vi "from string.vi"(8 "error in":errorcluster, 9 "channel data":string, 10 "identifier":string, 11 "channel in":refnum<class "fpga channel.lvclass">) -> (0 "error out":errorcluster, 3 "channel out":refnum<class "fpga channel.lvclass">)   [LabVIEW 2015, in "fpga channel.lvclass"]
uses:
  fpga channel.lvclass
  fpga channel.lvclass/fpga channel.ctl
  Read FXP type.vi
  Write FXP type.vi
  <vilib>/NI/Tag Bus Module Framework/channel/TBM channel.lvclass
  <vilib>/NI/Configuration Framework/serializable configuration/NISE_CEF_serializable configuration.lvclass
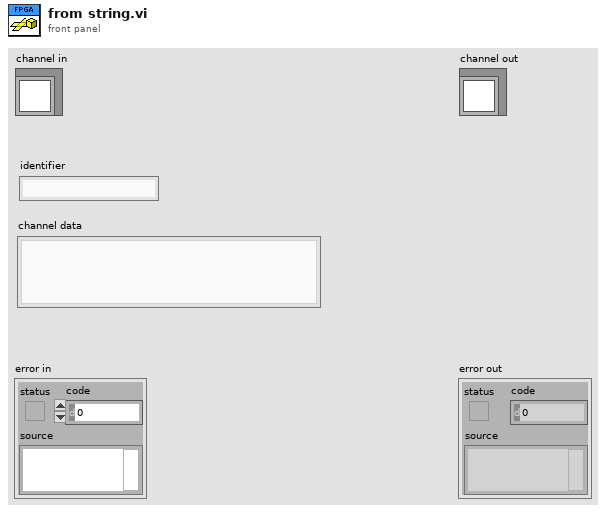
[diagram p1: front panel]
types:
  T1 = typedef "LVFixedPointRepBitsTypeDef.ctl" = cluster{"Signed":bool, "Word Length":u32, "Integer Word Length":i32}
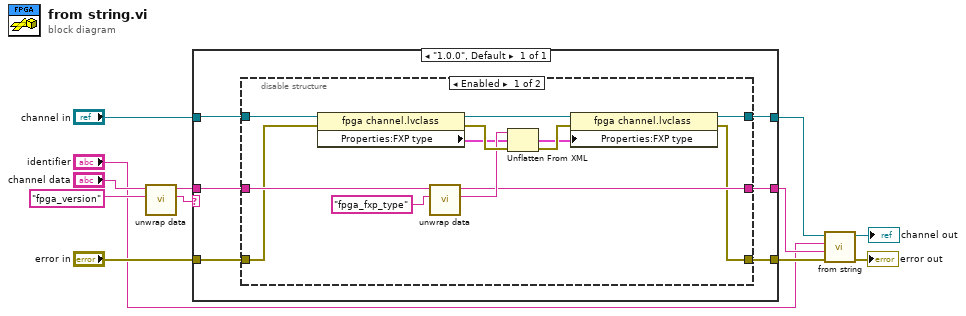
[diagram p0: block diagram]
diagram:
  n1 = call <vilib>:"unwrap data.vi"("identifier"="fpga_version", "data to unwrap"="channel data") -> ("unwrapped data"=w6:string, "remaining string"=w7:string)  [unwired: 8 in]
  n2 = case shown="\"1.0.0\", Default" w6 {
    tunnel: "error in" -> [w15]
    tunnel: w7 -> [w17]
    tunnel: "channel in" -> [w14]
    tunnel: [w18] -> w4
    tunnel: [w16] -> w3
    tunnel: [w13] -> w2
    frame "1.0.0", Default {
      n3 = disable-structure shown="Enabled" {
        disable-tunnel: [w29 w34] -> w18
        disable-tunnel: w17 -> [w28 w33]
        disable-tunnel: [w25 w33] -> w16
        disable-tunnel: w15 -> [w22 w32]
        disable-tunnel: w14 -> [w21 w34]
        disable-tunnel: [w19 w32] -> w13
        frame Enabled {
          n4 = property class="fpga channel.lvclass"(reference=w21, error in=w22) -> (reference out=w20:refnum<class "fpga channel.lvclass">, error out=w31:errorcluster, "Properties:FXP type"=w23:T1)
          n5 = call <vilib>:"unwrap data.vi"("identifier"="fpga_fxp_type" ("additional identifier"), "data to unwrap"=w28) -> ("unwrapped data"=w26:string, "remaining string"=w25:string)  [unwired: 8 in]
          n6 = Unflatten From XML(xml string=w26, type=w23, error in (no error)=w31) -> (value=w24:T1, error out=w30:errorcluster)
          n7 = property class="fpga channel.lvclass"(reference=w20, error in=w30, "Properties:FXP type"=w24) -> (reference out=w29:refnum<class "fpga channel.lvclass">, error out=w19:errorcluster)
        }
        frame Disabled {
        }
      }
    }
  }
  n8 = call-parent "from string.vi"("error in"=w2, "channel data"=w3, "identifier"="identifier", "channel in"=w4) -> ("error out"=→"error out":errorcluster, "channel out"=→"channel out":refnum<class "fpga channel.lvclass">)  [unwired: 6 in]
